vi "Control Documentation Tool.vi"() -> ()   [LabVIEW 2012]
uses:
  <vilib>/regexp/Match Regular Expression.xnode
panel:
  in  "Write Values":bool
  in  "File Path Control":path=path "C:/Users/husmith/Documents/Hunter Drive/minisystemtracking.1/iWorx/Code"
  in  "Documentation":T1(array[cluster])=[{"Control Name"="Autoscale Y", "Tip Strip"="Auto Tip", "Description"="Auto Description!"}, {"Control Name"="Clear Chart", "Tip Strip"="Clear Tip", "Description"="Clear Description"}, {"Control Name"="Set SP1", "Tip Strip"="", "Description"=""}, {"Control Name"="Set SP2", "Tip Strip"="", "Description"=""}, {"Control Name"="Pause", "Tip Strip"="", "Description"=""}, {"Control Name"="Open Log", "Tip Strip"="", "Description"=""}, {"Control Name"="Snapshot", "Tip Strip"="", "Description"=""}, {"Control Name"="stop", "Tip Strip"="", "Description"=""}, {"Control Name"="Set Up", "Tip Strip"="", "Description"=""}, {"Control Name"="Raw Signal", "Tip Strip"="", "Description"=""}, {"Control Name"="Processed Signal", "Tip Strip"="", "Description"=""}, {"Control Name"="Channel", "Tip Strip"="", "Description"=""}, {"Control Name"="Sample Timing", "Tip Strip"="", "Description"=""}, {"Control Name"="Calibration Data", "Tip Strip"="", "Description"=""}]
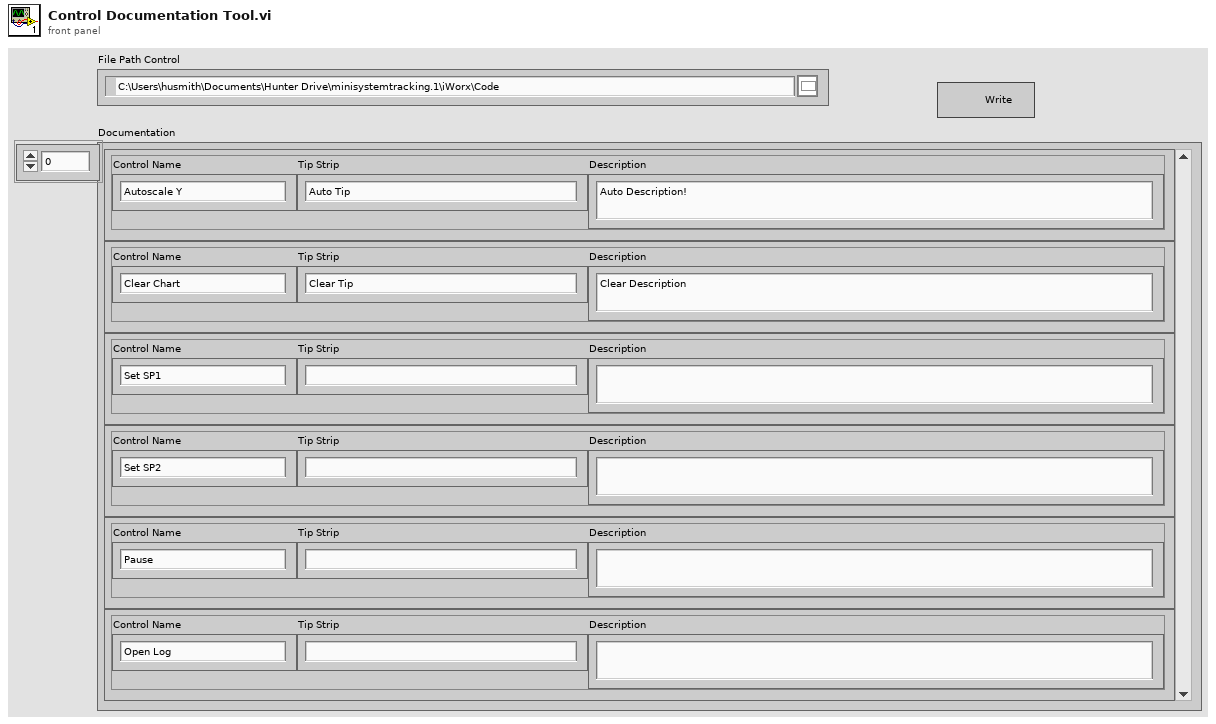
[diagram p1: front panel]
types:
  T1 = cluster{"Control Name":string, "Tip Strip":string, "Description":string}[]
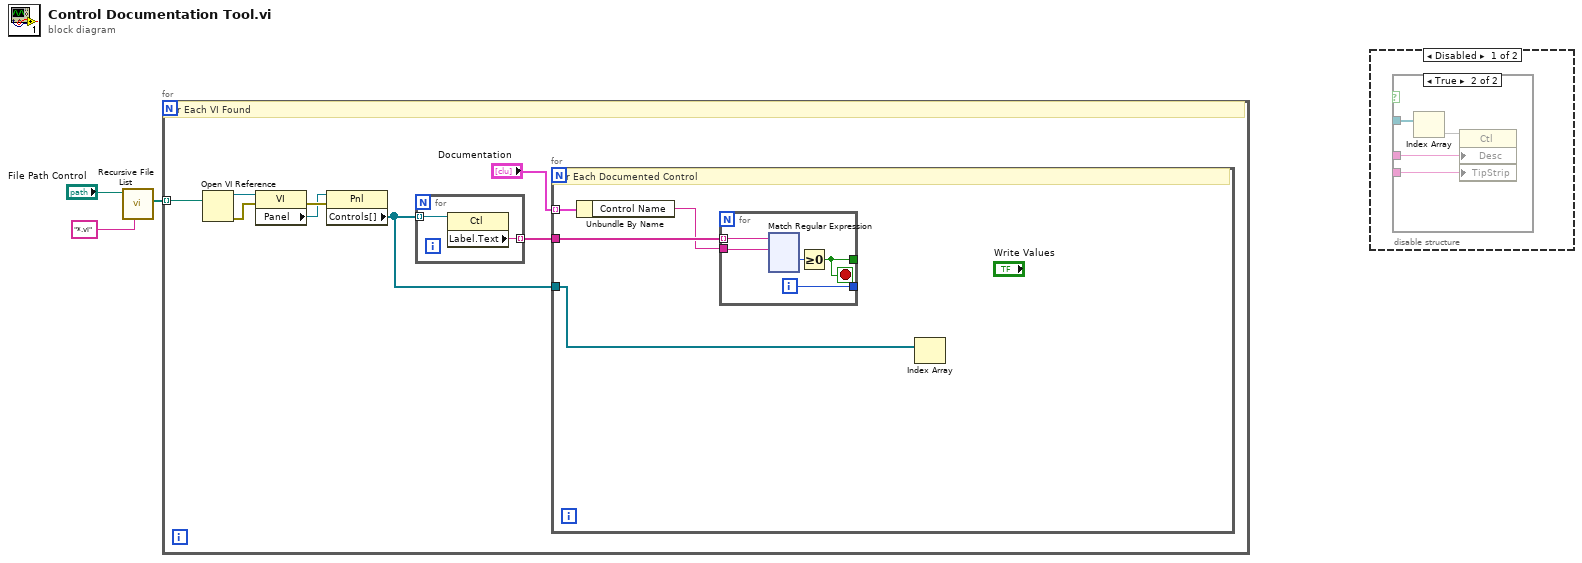
[diagram p0: block diagram]
diagram:
  n1 = call <vilib>:"Recursive File List.vi"("pattern"="*.vi", "Folder Path"="File Path Control") -> ("All Files in Dir"=w1:path[])  [unwired: 5 in, 4 out]
  n2 = for {
    tunnel: w1 -> [w5] mode=indexing
    # "For Each VI Found"
    n3 = Open VI Reference(vi path=w5) -> (vi reference=w4:refnum<vi>, error out=w10:errorcluster)  [unwired: 5 in]
    n4 = property on="Property Node" class="VI"(reference=w4, error in=w10) -> (error out=w9:errorcluster, "Panel"=w8:refnum<vi>)  [unwired: 1 out]
    n5 = property on="Property Node" class="Pnl"(reference=w8, error in=w9) -> ("Controls[]"=w6:refnum<vi>[])  [unwired: 2 out]
    n6 = for {
      tunnel: w6 -> [w13] mode=indexing
      tunnel: [w12] -> w7 mode=indexing
      n7 = property on="Property Node" class="Ctl"(reference=w13) -> ("Label.Text"=w12:string)  [unwired: 1 in, 2 out]
    }
    n8 = for {
      tunnel: "Documentation" -> [w17] mode=indexing
      tunnel: w7 -> [w16]
      tunnel: w6 -> [w14]
      # "For Each Documented Control"
      n9 = Unbundle By Name(w17) -> ("Control Name"=w15:string)
      n10 = for {
        tunnel: w16 -> [w22] mode=indexing
        tunnel: [w21] -> _
        tunnel: w15 -> [w20]
        tunnel: [w18] -> _
        i -> [w21]
        stop <- w18 stop-if-true
        n11 = xnode "Match Regular Expression"("input string"=w22, "regular expression"=w20) -> ("offset past match"=w19:i32)  [unwired: 4 in, 4 out]
        n12 = Greater Or Equal To 0?(x=w19) -> (x >= 0?=w18:bool)
      }
      n13 = Index Array(array=w14) -> ()  [unwired: 1 in, 1 out]
    }
  }
  n14 = disable-structure shown="Disabled" {
    frame Disabled {
      n15 = case shown="True" {
        selector: _ -> [_ _]
        tunnel: _ -> [_ w137]
        tunnel: _ -> [_ w135]
        tunnel: _ -> [_ w134]
        frame False {
        }
        frame True {
          n16 = Index Array(array=w137) -> (element=w136)  [unwired: 1 in]
          n17 = property on="Property Node" class="Ctl"(reference=w136, "Desc"=w135, "TipStrip"=w134) -> ()  [unwired: 1 in, 2 out]
        }
      }
    }
    frame Enabled {
    }
  }
